vi "Loader.vi"(11 "Robot_Interface":refnum<class "Robot_Interface.lvclass">) -> ()   [LabVIEW 2015, in "Robot_Interface.lvclass"]
uses:
  Robot_Interface.lvclass
  Robot_Interface.lvclass/Robot_Interface.ctl
panel:
  out "error out":errorcluster
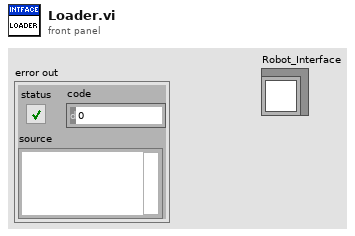
[diagram p1: front panel]
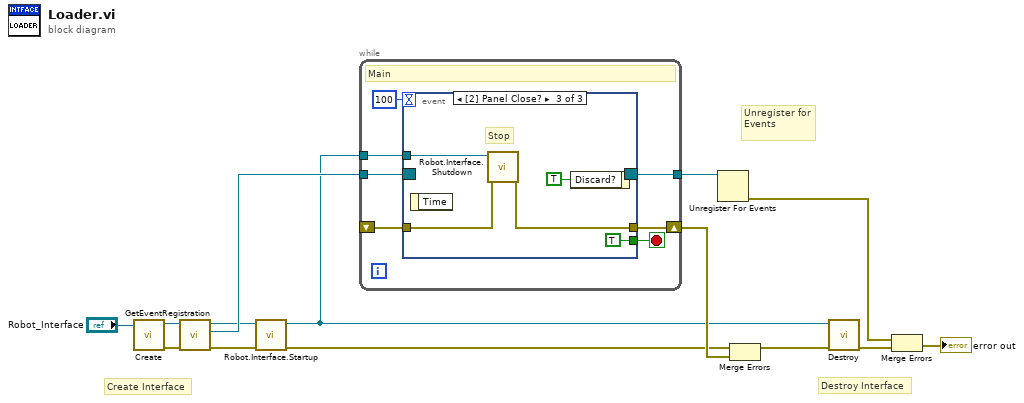
[diagram p0: block diagram]
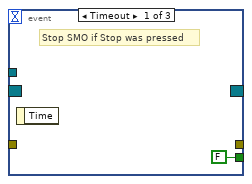
[diagram p2: hidden frame]
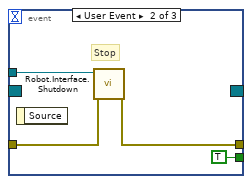
[diagram p3: hidden frame]
diagram:
  # "Create Interface"
  # "Destroy Interface"
  # "Unregister for Events"
  n1 = call-dynamic "Create.vi"("Robot_Interface in"="Robot_Interface") -> ("error out"=w10:errorcluster, "Robot_Interface out"=w7:refnum<class "Robot_Interface.lvclass">)  [unwired: 9 in]
  n2 = call "GetEventRegistration.vi"("error in (no error)"=w10, "Robot_Interface in"=w7) -> ("error out"=w5:errorcluster, "Shutdown"=w9:refnum<event-registration>, "Robot_Interface out"=w6:refnum<class "Robot_Interface.lvclass">)  [unwired: 7 in]
  n3 = call-dynamic "Robot.Interface.Startup.vi"("error in (no error)"=w5, "Robot_Interface in"=w6) -> ("error out"=w4:errorcluster, "Robot_Interface out"=w3:refnum<class "Robot_Interface.lvclass">)  [unwired: 8 in]
  n4 = while {
    shift-right: [w20] -> w14
    shift-left: _ -> [w19]
    tunnel: w9 -> [w18]
    tunnel: [w17] -> w11
    tunnel: w3 -> [w16]
    stop <- w21 stop-if-true
    # "Main"
    n5 = event shown="[2] Panel Close?" {
      selector: w18 -> [_ _ _]
      dyn-events: [_ _ _] -> w17
      timeout: 100 -> [_ _ _]
      tunnel: [FALSE ("Stop") TRUE ("Stop") TRUE ("Stop")] -> w21
      tunnel: w16 -> [_ w26 w31]
      tunnel: [_ w24 w29] -> w20
      tunnel: w19 -> [_ w25 w30]
      event Timeout {
        # "Stop SMO if Stop was pressed"
        n6 = event-data() -> ()  [unwired: 1 in, 1 out]
      }
      event User Event {
        # "Stop"
        n7 = event-data() -> ()  [unwired: 1 in, 1 out]
        n8 = call-dynamic "Robot.Interface.Shutdown.vi"("error in (no error)"=w25, "Robot_Interface in"=w26) -> ("error out"=w24:errorcluster)  [unwired: 8 in, 1 out]
      }
      event Panel Close? {
        # "Stop"
        n9 = event-data() -> ()  [unwired: 1 in, 1 out]
        n10 = call-dynamic "Robot.Interface.Shutdown.vi"("error in (no error)"=w30, "Robot_Interface in"=w31) -> ("error out"=w29:errorcluster)  [unwired: 8 in, 1 out]
        n11 = event-data("Discard?"=TRUE) -> ()  [unwired: 1 in, 1 out]
      }
    }
  }
  n12 = Unregister For Events(event registration refnum=w11) -> (error out=w12:errorcluster)  [unwired: 1 in]
  n13 = Merge Errors(w4, w14) -> (w8:errorcluster)
  n14 = call-dynamic "Destroy.vi"("error in (no error)"=w8, "Robot_Interface in"=w3) -> ("error out"=w2:errorcluster)  [unwired: 8 in, 1 out]
  n15 = Merge Errors(w12, w2) -> (→"error out":errorcluster)
